vi "Dresden Edit Recipe(in).vi"() -> ()   [LabVIEW 2009] (continued)
            n1177 = local read "R Cmb Step3 Coating Power Active"() -> (w886:bool)
            n1178 = local read "R Cmb Step4 Coating Power Active"() -> (w885:bool)
            n1179 = local read "R Cmb Step5 Coating Power Active"() -> (w884:bool)
            n1180 = local read "R Cmb Step6 Coating Power Active"() -> (w883:bool)
            n1181 = local read "R Cmb Step7 Coating Power Active"() -> (w882:bool)
            n1182 = local read "R Cmb Step8 Coating Power Active"() -> (w881:bool)
            n1183 = local read "R Cmb Step9 Coating Power Active"() -> (w880:bool)
            n1184 = local read "R Cmb Step10 Coating Power Active"() -> (w879:bool)
            n1185 = local read "R Single RF Step6 Coating Power Active"() -> (w835:bool)
            n1186 = local read "R Cmb Interval length 1"() -> (w889:dbl)
            n1187 = Equal?(x=w1001, y=1) -> (x = y?=w999:bool)
            n1188 = case shown="False" w999 {
              frame #0 {
                w2466 = T5."Disabled and Grayed Out" ("Disabled")
                w2467 = 0.0 ("R Cmb Ch2 DC Ignition Power")
                w2468 = FALSE ("R Cmb Ch2 DC Target Clean Power Active")
                w2469 = ""
                n1189 = local write "R Cmb Number of cycle"(w2467) -> ()
                n1190 = local write "R Cmb Interval length 6"(w2467) -> ()
                n1191 = local write "R Cmb Interval length 7"(w2467) -> ()
                n1192 = local write "R Cmb Interval length 8"(w2467) -> ()
                n1193 = local write "R Cmb Interval length 9"(w2467) -> ()
                n1194 = local write "R Cmb Interval length 10"(w2467) -> ()
                n1195 = local write "R Cmb Ch2 Step6 Coating Power"(w2467) -> ()
                n1196 = local write "R Cmb Ch2 Step7 Coating Power"(w2467) -> ()
                n1197 = local write "R Cmb Ch2 Step8 Coating Power"(w2467) -> ()
                n1198 = local write "R Cmb Ch2 Step9 Coating Power"(w2467) -> ()
                n1199 = local write "R Cmb Ch2 Step10 Coating Power"(w2467) -> ()
                n1200 = local write "R Cmb Interval length 6"(w2467) -> ()
                n1201 = local write "R Cmb Interval length 7"(w2467) -> ()
                n1202 = local write "R Cmb Interval length 8"(w2467) -> ()
                n1203 = local write "R Cmb Interval length 9"(w2467) -> ()
                n1204 = local write "R Cmb Interval length 10"(w2467) -> ()
                n1205 = local write "R Cmb Interval length 1"(w2467) -> ()
                n1206 = local write "R Cmb Interval length 2"(w2467) -> ()
                n1207 = local write "R Cmb Interval length 3"(w2467) -> ()
                n1208 = local write "R Cmb Interval length 4"(w2467) -> ()
                n1209 = local write "R Cmb Interval length 5"(w2467) -> ()
                n1210 = local write "R Cmb Interval length 2"(w2467) -> ()
                n1211 = local write "R Cmb Interval length 3"(w2467) -> ()
                n1212 = local write "R Cmb Interval length 4"(w2467) -> ()
                n1213 = local write "R Cmb Interval length 5"(w2467) -> ()
                n1214 = local write "R Cmb Ch2 Step1 Coating Power"(w2467) -> ()
                n1215 = local write "R Cmb Ch2 Step2 Coating Power"(w2467) -> ()
                n1216 = local write "R Cmb Ch2 Step3 Coating Power"(w2467) -> ()
                n1217 = local write "R Cmb Ch2 Step4 Coating Power"(w2467) -> ()
                n1218 = local write "R Cmb Ch2 Step5 Coating Power"(w2467) -> ()
                n1219 = local write "R Cmb Ch3 Step1 Coating Power"(w2467) -> ()
                n1220 = local write "R Cmb Step6 Coating Power Active"(w2468) -> ()
                n1221 = local write "R Cmb Step7 Coating Power Active"(w2468) -> ()
                n1222 = local write "R Cmb Step8 Coating Power Active"(w2468) -> ()
                n1223 = local write "R Cmb Step9 Coating Power Active"(w2468) -> ()
                n1224 = local write "R Cmb Step10 Coating Power Active"(w2468) -> ()
                n1225 = local write "R Cmb Step1 Coating Power Active"(w2468) -> ()
                n1226 = local write "R Cmb Step2 Coating Power Active"(w2468) -> ()
                n1227 = local write "R Cmb Step3 Coating Power Active"(w2468) -> ()
                n1228 = local write "R Cmb Step4 Coating Power Active"(w2468) -> ()
                n1229 = local write "R Cmb Step5 Coating Power Active"(w2468) -> ()
                n1230 = local write "R Cmb Ch2 Target material"(w2469) -> ()
                n1231 = local write "R Cmb Ch3 Target material"(w2469) -> ()
                n1232 = property on="R Cmb Number of cycle" class="DigNum (strict)"("DisabledEnum"=w2466) -> ()  [unwired: 2 in, 2 out]
                n1233 = property on="R Cmb Ch2 Step1 Coating Power" class="DigNum (strict)"("DisabledEnum"=w2466) -> ()  [unwired: 2 in, 2 out]
                n1234 = property on="R Cmb Ch2 Step2 Coating Power" class="DigNum (strict)"("DisabledEnum"=w2466) -> ()  [unwired: 2 in, 2 out]
                n1235 = property on="R Cmb Ch2 Step3 Coating Power" class="DigNum (strict)"("DisabledEnum"=w2466) -> ()  [unwired: 2 in, 2 out]
                n1236 = property on="R Cmb Ch2 Step4 Coating Power" class="DigNum (strict)"("DisabledEnum"=w2466) -> ()  [unwired: 2 in, 2 out]
                n1237 = property on="R Cmb Ch2 Step5 Coating Power" class="DigNum (strict)"("DisabledEnum"=w2466) -> ()  [unwired: 2 in, 2 out]
                n1238 = property on="R Cmb Ch2 Step6 Coating Power" class="DigNum (strict)"("DisabledEnum"=w2466) -> ()  [unwired: 2 in, 2 out]
                n1239 = property on="R Cmb Ch2 Step7 Coating Power" class="DigNum (strict)"("DisabledEnum"=w2466) -> ()  [unwired: 2 in, 2 out]
                n1240 = property on="R Cmb Ch2 Step8 Coating Power" class="DigNum (strict)"("DisabledEnum"=w2466) -> ()  [unwired: 2 in, 2 out]
                n1241 = property on="R Cmb Ch2 Step9 Coating Power" class="DigNum (strict)"("DisabledEnum"=w2466) -> ()  [unwired: 2 in, 2 out]
                n1242 = property on="R Cmb Ch2 Step10 Coating Power" class="DigNum (strict)"("DisabledEnum"=w2466) -> ()  [unwired: 2 in, 2 out]
                n1243 = property on="R Cmb Ch3 Step1 Coating Power" class="DigNum (strict)"("DisabledEnum"=w2466) -> ()  [unwired: 2 in, 2 out]
                n1244 = property on="R Cmb Ch3 Step2 Coating Power" class="DigNum (strict)"("DisabledEnum"=w2466) -> ()  [unwired: 2 in, 2 out]
                n1245 = property on="R Cmb Ch3 Step3 Coating Power" class="DigNum (strict)"("DisabledEnum"=w2466) -> ()  [unwired: 2 in, 2 out]
                n1246 = property on="R Cmb Ch3 Step4 Coating Power" class="DigNum (strict)"("DisabledEnum"=w2466) -> ()  [unwired: 2 in, 2 out]
                n1247 = property on="R Cmb Ch3 Step5 Coating Power" class="DigNum (strict)"("DisabledEnum"=w2466) -> ()  [unwired: 2 in, 2 out]
                n1248 = property on="R Cmb Ch3 Step6 Coating Power" class="DigNum (strict)"("DisabledEnum"=w2466) -> ()  [unwired: 2 in, 2 out]
                n1249 = property on="R Cmb Ch3 Step7 Coating Power" class="DigNum (strict)"("DisabledEnum"=w2466) -> ()  [unwired: 2 in, 2 out]
                n1250 = property on="R Cmb Ch3 Step8 Coating Power" class="DigNum (strict)"("DisabledEnum"=w2466) -> ()  [unwired: 2 in, 2 out]
                n1251 = property on="R Cmb Ch3 Step9 Coating Power" class="DigNum (strict)"("DisabledEnum"=w2466) -> ()  [unwired: 2 in, 2 out]
                n1252 = property on="R Cmb Ch3 Step10 Coating Power" class="DigNum (strict)"("DisabledEnum"=w2466) -> ()  [unwired: 2 in, 2 out]
                n1253 = property on="R Cmb Interval length 10" class="DigNum (strict)"("DisabledEnum"=w2466) -> ()  [unwired: 2 in, 2 out]
                n1254 = property on="R Cmb Interval length 6" class="DigNum (strict)"("DisabledEnum"=w2466) -> ()  [unwired: 2 in, 2 out]
                n1255 = property on="R Cmb Interval length 7" class="DigNum (strict)"("DisabledEnum"=w2466) -> ()  [unwired: 2 in, 2 out]
                n1256 = property on="R Cmb Interval length 8" class="DigNum (strict)"("DisabledEnum"=w2466) -> ()  [unwired: 2 in, 2 out]
                n1257 = property on="R Cmb Interval length 9" class="DigNum (strict)"("DisabledEnum"=w2466) -> ()  [unwired: 2 in, 2 out]
                n1258 = property on="R Cmb Interval length 1" class="DigNum (strict)"("DisabledEnum"=w2466) -> ()  [unwired: 2 in, 2 out]
                n1259 = property on="R Cmb Interval length 2" class="DigNum (strict)"("DisabledEnum"=w2466) -> ()  [unwired: 2 in, 2 out]
                n1260 = property on="R Cmb Interval length 3" class="DigNum (strict)"("DisabledEnum"=w2466) -> ()  [unwired: 2 in, 2 out]
                n1261 = property on="R Cmb Interval length 4" class="DigNum (strict)"("DisabledEnum"=w2466) -> ()  [unwired: 2 in, 2 out]
                n1262 = property on="R Cmb Interval length 5" class="DigNum (strict)"("DisabledEnum"=w2466) -> ()  [unwired: 2 in, 2 out]
              }
              frame #1 {
                w2471 = T5."Disabled and Grayed Out" ("Disabled")
                n1263 = property on="R Single DC Interval length1" class="DigNum (strict)"("DisabledEnum"=w2471) -> ()  [unwired: 2 in, 2 out]
                n1264 = property on="R Single DC Step1 Coating Power" class="DigNum (strict)"("DisabledEnum"=w2471) -> ()  [unwired: 2 in, 2 out]
                n1265 = property on="R Cmb Number of cycle" class="DigNum (strict)"("DisabledEnum"=T5."Enabled" ("Disabled")) -> ()  [unwired: 2 in, 2 out]
                n1266 = local write "R Single DC Step1 Coating Power Active"(FALSE ("R Single DC Step1 Coating Power Active")) -> ()
                n1267 = local write "R Cmb Step1 Coating Power Active"(TRUE ("R Cmb Ch2 Step1 Coating Power Active")) -> ()
                n1268 = property on="R Single DC Target material" class="Str"("DisabledEnum"=T5."Disabled and Grayed Out" ("Disabled")) -> ()  [unwired: 2 in, 2 out]
              }
            }
            n1269 = case shown="True" w1011 {
              frame #0 {
                w2495 = T5."Disabled and Grayed Out" ("Disabled")
                w2494 = 0.0 ("R DC Ignition Power")
                w2493 = FALSE ("R DC Target Clean")
                n1270 = local write "R Single RF Interval length10"(w2494) -> ()
                n1271 = local write "R Single RF Interval length"(w2494) -> ()
                n1272 = local write "R Single RF Ramp up Time"(w2494) -> ()
                n1273 = local write "R Single RF  Step1 Coating Power"(w2494) -> ()
                n1274 = local write "R Single RF Step2 Coating Power"(w2494) -> ()
                n1275 = local write "R Single RF Step3 Coating Power"(w2494) -> ()
                n1276 = local write "R Single RF Step4 Coating Power"(w2494) -> ()
                n1277 = local write "R Single RF Step5 Coating Power"(w2494) -> ()
                n1278 = local write "R Single RF Ramp down Time"(w2494) -> ()
                n1279 = local write "R Single RF Interval length9"(w2494) -> ()
                n1280 = local write "R Single RF Interval length6"(w2494) -> ()
                n1281 = local write "R Single RF Target material"("") -> ()
                n1282 = local write "R Single RF Ramp up"(w2493) -> ()
                n1283 = local write "R Single RF Ramp down"(w2493) -> ()
                n1284 = local write "R Single RF Step1 Coating Power Active"(w2493) -> ()
                n1285 = local write "R Single RF Step2 Coating Power Active"(w2493) -> ()
                n1286 = local write "R Single RF Step3 Coating Power Active"(w2493) -> ()
                n1287 = local write "R Single RF Step4 Coating Power Active"(w2493) -> ()
                n1288 = local write "R Single RF Step5 Coating Power Active"(w2493) -> ()
                n1289 = local write "R Single RF Interval length8"(w2494) -> ()
                n1290 = local write "R Single RF Interval length7"(w2494) -> ()
                n1291 = local write "R Single RF Step6 Coating Power"(w2494) -> ()
                n1292 = local write "R Single RF Step7 Coating Power"(w2494) -> ()
                n1293 = local write "R Single RF Step8 Coating Power"(w2494) -> ()
                n1294 = local write "R Single RF Step9 Coating Power"(w2494) -> ()
                n1295 = local write "R Single RF Step10 Coating Power"(w2494) -> ()
                n1296 = local write "R Single RF Interval length2"(w2494) -> ()
                n1297 = local write "R Single RF Interval length3"(w2494) -> ()
                n1298 = local write "R Single RF Interval length4"(w2494) -> ()
                n1299 = local write "R Single RF Interval length5"(w2494) -> ()
                n1300 = local write "R Single RF Step6 Coating Power Active"(w2493) -> ()
                n1301 = local write "R Single RF Step7 Coating Power Active"(w2493) -> ()
                n1302 = local write "R Single RF Step8 Coating Power Active"(w2493) -> ()
                n1303 = local write "R Single RF Step9 Coating Power Active"(w2493) -> ()
                n1304 = local write "R Single RF Step10 Coating Power Active"(w2493) -> ()
                n1305 = property on="R Single RF Interval length" class="DigNum (strict)"("DisabledEnum"=w2495) -> ()  [unwired: 2 in, 2 out]
                n1306 = property on="R Single RF Step6 Coating Power" class="DigNum (strict)"("DisabledEnum"=w2495) -> ()  [unwired: 2 in, 2 out]
                n1307 = property on="R Single RF Step7 Coating Power" class="DigNum (strict)"("DisabledEnum"=w2495) -> ()  [unwired: 2 in, 2 out]
                n1308 = property on="R Single RF Step8 Coating Power" class="DigNum (strict)"("DisabledEnum"=w2495) -> ()  [unwired: 2 in, 2 out]
                n1309 = property on="R Single RF Step9 Coating Power" class="DigNum (strict)"("DisabledEnum"=w2495) -> ()  [unwired: 2 in, 2 out]
                n1310 = property on="R Single RF Step10 Coating Power" class="DigNum (strict)"("DisabledEnum"=w2495) -> ()  [unwired: 2 in, 2 out]
                n1311 = property on="R Single RF Interval length2" class="DigNum (strict)"("DisabledEnum"=w2495) -> ()  [unwired: 2 in, 2 out]
                n1312 = property on="R Single RF Interval length3" class="DigNum (strict)"("DisabledEnum"=w2495) -> ()  [unwired: 2 in, 2 out]
                n1313 = property on="R Single RF Interval length4" class="DigNum (strict)"("DisabledEnum"=w2495) -> ()  [unwired: 2 in, 2 out]
                n1314 = property on="R Single RF Interval length5" class="DigNum (strict)"("DisabledEnum"=w2495) -> ()  [unwired: 2 in, 2 out]
                n1315 = property on="R Single RF Interval length6" class="DigNum (strict)"("DisabledEnum"=w2495) -> ()  [unwired: 2 in, 2 out]
                n1316 = property on="R Single RF Ramp up Time" class="DigNum (strict)"("DisabledEnum"=w2495) -> ()  [unwired: 2 in, 2 out]
                n1317 = property on="R Single RF  Step1 Coating Power" class="DigNum (strict)"("DisabledEnum"=w2495) -> ()  [unwired: 2 in, 2 out]
                n1318 = property on="R Single RF Step2 Coating Power" class="DigNum (strict)"("DisabledEnum"=w2495) -> ()  [unwired: 2 in, 2 out]
                n1319 = property on="R Single RF Step3 Coating Power" class="DigNum (strict)"("DisabledEnum"=w2495) -> ()  [unwired: 2 in, 2 out]
                n1320 = property on="R Single RF Step4 Coating Power" class="DigNum (strict)"("DisabledEnum"=w2495) -> ()  [unwired: 2 in, 2 out]
                n1321 = property on="R Single RF Step5 Coating Power" class="DigNum (strict)"("DisabledEnum"=w2495) -> ()  [unwired: 2 in, 2 out]
                n1322 = property on="R Single RF Ramp down Time" class="DigNum (strict)"("DisabledEnum"=w2495) -> ()  [unwired: 2 in, 2 out]
                n1323 = property on="R Single RF Interval length10" class="DigNum (strict)"("DisabledEnum"=w2495) -> ()  [unwired: 2 in, 2 out]
                n1324 = property on="R Single RF Interval length9" class="DigNum (strict)"("DisabledEnum"=w2495) -> ()  [unwired: 2 in, 2 out]
                n1325 = property on="R Single RF Interval length7" class="DigNum (strict)"("DisabledEnum"=w2495) -> ()  [unwired: 2 in, 2 out]
                n1326 = property on="R Single RF Interval length8" class="DigNum (strict)"("DisabledEnum"=w2495) -> ()  [unwired: 2 in, 2 out]
              }
              frame #1 {
                n1327 = local write "R Single RF Step1 Coating Power Active"(TRUE ("R Single RF Step1 Coating Power Active")) -> ()
                n1328 = local write "R Set Pressure mtorr"(0.001 ("R Set Pressure mtorr")) -> ()
              }
            }
            n1329 = local read "R Single DC Step5 Coating Power Active"() -> (w846:bool)
            n1330 = case shown="True" w1016 {
              frame #0 {
                w2499 = 0.0 ("R_Microwave Power")
                w2500 = T5."Enabled" ("Disabled")
                n1331 = property on="R Argon Flow sccm" class="DigNum (strict)"("DisabledEnum"=w2500) -> ()  [unwired: 2 in, 2 out]
                n1332 = property on="R Set Pressure mtorr" class="DigNum (strict)"("DisabledEnum"=w2500) -> ()  [unwired: 2 in, 2 out]
                n1333 = local write "R_Single Microwave Power"(w2499) -> ()
                n1334 = local write "R_Single Microwave Time"(w2499) -> ()
                n1335 = property on="R_Single Microwave Power" class="DigNum (strict)"("DisabledEnum"=T5."Disabled and Grayed Out" ("Disabled")) -> ()  [unwired: 2 in, 2 out]
                n1336 = local write "R Single Pass Number"(w2499) -> ()
              }
              frame #1 {
                w2509 = T5."Disabled and Grayed Out" ("Disabled")
                n1337 = property on="R Set Pressure mtorr" class="DigNum (strict)"("DisabledEnum"=w2509) -> ()  [unwired: 2 in, 2 out]
                n1338 = property on="R Argon Flow sccm" class="DigNum (strict)"("DisabledEnum"=w2509) -> ()  [unwired: 2 in, 2 out]
                n1339 = local read "R Single Pass Number"() -> (w2507:dbl)
                n1340 = property on="R_Single Microwave Power" class="DigNum (strict)"("DisabledEnum"=T5."Enabled" ("Disabled")) -> ()  [unwired: 2 in, 2 out]
                n1341 = local write "R Argon Flow sccm"(200.0 ("R Argon Flow sccm")) -> ()
                n1342 = local write "R Set Pressure mtorr"(0.011 ("R Set Pressure mtorr")) -> ()
                n1343 = Less Or Equal?(x=w2507, y=1.5) -> (x <= y?=w2505:bool)
                n1344 = Select(t=1, s=w2505, f=2) -> (s? t:f=w2502:i32)
                n1345 = local write "R Single Pass Number"(w2502) -> ()
              }
            }
            n1346 = case shown="True" w1013 {
              frame #0 {
                w2487 = T5."Disabled and Grayed Out" ("Disabled")
                w2488 = 0.0 ("R DC Ignition Power")
                w2489 = FALSE ("R DC Target Clean")
                n1347 = local write "R Single DC Step1 Coating Power Active"(w2489) -> ()
                n1348 = local write "R Single DC Step2 Coating Power Active"(w2489) -> ()
                n1349 = local write "R Single DC Step3 Coating Power Active"(w2489) -> ()
                n1350 = local write "R Single DC Step4 Coating Power Active"(w2489) -> ()
                n1351 = local write "R Single DC Step5 Coating Power Active"(w2489) -> ()
                n1352 = local write "R Single DC Step6 Coating Power Active"(w2489) -> ()
                n1353 = local write "R Single DC Step7 Coating Power Active"(w2489) -> ()
                n1354 = local write "R Single DC Step8 Coating Power Active"(w2489) -> ()
                n1355 = local write "R Single DC Step9 Coating Power Active"(w2489) -> ()
                n1356 = local write "R Single DC Step10 Coating Power Active"(w2489) -> ()
                n1357 = local write "R_Single DC_Material ok"(w2489) -> ()
                n1358 = local write "R Single DC Target material"("") -> ()
                n1359 = local write "R Single DC Interval length1"(w2488) -> ()
                n1360 = local write "R Single DC Step1 Coating Power"(w2488) -> ()
                n1361 = local write "R Single DC Step2 Coating Power"(w2488) -> ()
                n1362 = local write "R Single DC Step3 Coating Power"(w2488) -> ()
                n1363 = local write "R Single DC Step4 Coating Power"(w2488) -> ()
                n1364 = local write "R Single DC Step5 Coating Power"(w2488) -> ()
                n1365 = local write "R Single DC Interval length2"(w2488) -> ()
                n1366 = local write "R Single DC Interval length3"(w2488) -> ()
                n1367 = local write "R Single DC Interval length4"(w2488) -> ()
                n1368 = local write "R Single DC Interval length5"(w2488) -> ()
                n1369 = local write "R Single DC Interval length6"(w2488) -> ()
                n1370 = local write "R Single DC Interval length7"(w2488) -> ()
                n1371 = local write "R Single DC Interval length8"(w2488) -> ()
                n1372 = local write "R Single DC Interval length9"(w2488) -> ()
                n1373 = local write "R Single DC Interval length10"(w2488) -> ()
                n1374 = property on="R Single DC Step6 Coating Power" class="DigNum (strict)"("DisabledEnum"=w2487) -> ()  [unwired: 2 in, 2 out]
                n1375 = property on="R Single DC Step7 Coating Power" class="DigNum (strict)"("DisabledEnum"=w2487) -> ()  [unwired: 2 in, 2 out]
                n1376 = property on="R Single DC Interval length6" class="DigNum (strict)"("DisabledEnum"=w2487) -> ()  [unwired: 2 in, 2 out]
                n1377 = property on="R Single DC Step1 Coating Power" class="DigNum (strict)"("DisabledEnum"=w2487) -> ()  [unwired: 2 in, 2 out]
                n1378 = property on="R Single DC Step2 Coating Power" class="DigNum (strict)"("DisabledEnum"=w2487) -> ()  [unwired: 2 in, 2 out]
                n1379 = property on="R Single DC Step3 Coating Power" class="DigNum (strict)"("DisabledEnum"=w2487) -> ()  [unwired: 2 in, 2 out]
                n1380 = property on="R Single DC Step4 Coating Power" class="DigNum (strict)"("DisabledEnum"=w2487) -> ()  [unwired: 2 in, 2 out]
                n1381 = property on="R Single DC Step5 Coating Power" class="DigNum (strict)"("DisabledEnum"=w2487) -> ()  [unwired: 2 in, 2 out]
                n1382 = property on="R Single DC Interval length1" class="DigNum (strict)"("DisabledEnum"=w2487) -> ()  [unwired: 2 in, 2 out]
                n1383 = property on="R Single DC Step8 Coating Power" class="DigNum (strict)"("DisabledEnum"=w2487) -> ()  [unwired: 2 in, 2 out]
                n1384 = property on="R Single DC Step9 Coating Power" class="DigNum (strict)"("DisabledEnum"=w2487) -> ()  [unwired: 2 in, 2 out]
                n1385 = property on="R Single DC Step10 Coating Power" class="DigNum (strict)"("DisabledEnum"=w2487) -> ()  [unwired: 2 in, 2 out]
                n1386 = property on="R Single DC Interval length2" class="DigNum (strict)"("DisabledEnum"=w2487) -> ()  [unwired: 2 in, 2 out]
                n1387 = property on="R Single DC Interval length3" class="DigNum (strict)"("DisabledEnum"=w2487) -> ()  [unwired: 2 in, 2 out]
                n1388 = property on="R Single DC Interval length4" class="DigNum (strict)"("DisabledEnum"=w2487) -> ()  [unwired: 2 in, 2 out]
                n1389 = property on="R Single DC Interval length5" class="DigNum (strict)"("DisabledEnum"=w2487) -> ()  [unwired: 2 in, 2 out]
                n1390 = property on="R Single DC Interval length7" class="DigNum (strict)"("DisabledEnum"=w2487) -> ()  [unwired: 2 in, 2 out]
                n1391 = property on="R Single DC Interval length6" class="DigNum (strict)"("DisabledEnum"=w2487) -> ()  [unwired: 2 in, 2 out]
                n1392 = property on="R Single DC Interval length8" class="DigNum (strict)"("DisabledEnum"=w2487) -> ()  [unwired: 2 in, 2 out]
                n1393 = property on="R Single DC Interval length9" class="DigNum (strict)"("DisabledEnum"=w2487) -> ()  [unwired: 2 in, 2 out]
                n1394 = property on="R Single DC Interval length10" class="DigNum (strict)"("DisabledEnum"=w2487) -> ()  [unwired: 2 in, 2 out]
              }
              frame #1 {
                n1395 = local write "R Single DC Step1 Coating Power Active"(TRUE ("R Single DC Step1 Coating Power Active")) -> ()
                n1396 = local write "R Set Pressure mtorr"(0.004 ("R Set Pressure mtorr")) -> ()
              }
            }
            n1397 = local read "R Single RF Step7 Coating Power Active"() -> (w834:bool)
            n1398 = local read "R Single DC Step6 Coating Power Active"() -> (w845:bool)
            n1399 = Boolean To (0,1)(Boolean=w890) -> (0, 1=w900:i16)
            n1400 = case shown="False" w842 {
              frame #0 {
                n1401 = local write "R Single DC Step10 Coating Power Active"(FALSE ("R Single DC Step8 Coating Power Active")) -> ()
              }
              frame #1 {
                n1402 = local read "R Single DC Step10 Coating Power Active"() -> (w1118:bool)
                n1403 = case shown="False" w1118 {
                  frame #0 {
                    w1119 = 0.0 ("R Single DC Step10 Coating Power")
                    w1120 = T5."Disabled and Grayed Out" ("Disabled")
                    n1404 = local write "R Single DC Step10 Coating Power"(w1119) -> ()
                    n1405 = local write "R Single DC Interval length10"(w1119) -> ()
                    n1406 = property on="R Single DC Step10 Coating Power" class="DigNum (strict)"("DisabledEnum"=w1120) -> ()  [unwired: 2 in, 2 out]
                    n1407 = property on="R Single DC Interval length10" class="DigNum (strict)"("DisabledEnum"=w1120) -> ()  [unwired: 2 in, 2 out]
                  }
                  frame #1 {
                    w1121 = T5."Enabled" ("Disabled")
                    n1408 = property on="R Single DC Step10 Coating Power" class="DigNum (strict)"("DisabledEnum"=w1121) -> ()  [unwired: 2 in, 2 out]
                    n1409 = property on="R Single DC Interval length10" class="DigNum (strict)"("DisabledEnum"=w1121) -> ()  [unwired: 2 in, 2 out]
                  }
                }
              }
            }
            n1410 = case shown="False" w843 {
              frame #0 {
                w1122 = FALSE ("R Single DC Step8 Coating Power Active")
                n1411 = local write "R Single DC Step10 Coating Power Active"(w1122) -> ()
                n1412 = local write "R Single DC Step9 Coating Power Active"(w1122) -> ()
              }
              frame #1 {
                n1413 = local read "R Single DC Step9 Coating Power Active"() -> (w1123:bool)
                n1414 = case shown="False" w1123 {
                  frame #0 {
                    w1124 = 0.0 ("R Single DC Step9 Coating Power")
                    w1125 = T5."Disabled and Grayed Out" ("Disabled")
                    n1415 = property on="R Single DC Step9 Coating Power" class="DigNum (strict)"("DisabledEnum"=w1125) -> ()  [unwired: 2 in, 2 out]
                    n1416 = property on="R Single DC Interval length9" class="DigNum (strict)"("DisabledEnum"=w1125) -> ()  [unwired: 2 in, 2 out]
                    n1417 = local write "R Single DC Step9 Coating Power"(w1124) -> ()
                    n1418 = local write "R Single DC Interval length9"(w1124) -> ()
                  }
                  frame #1 {
                    w1126 = T5."Enabled" ("Disabled")
                    n1419 = property on="R Single DC Interval length9" class="DigNum (strict)"("DisabledEnum"=w1126) -> ()  [unwired: 2 in, 2 out]
                    n1420 = property on="R Single DC Step9 Coating Power" class="DigNum (strict)"("DisabledEnum"=w1126) -> ()  [unwired: 2 in, 2 out]
                  }
                }
              }
            }
            n1421 = local read "R Cmb Interval length 9"() -> (w872:dbl)
            n1422 = local read "R Cmb Interval length 3"() -> (w878:dbl)
            n1423 = local read "R Cmb Interval length 4"() -> (w877:dbl)
            n1424 = local read "R Cmb Interval length 10"() -> (w871:dbl)
            n1425 = local read "R Cmb Interval length 2"() -> (w887:dbl)
            n1426 = local read "R Cmb Interval length 5"() -> (w876:dbl)
            n1427 = case shown="True" w988 {
              frame #0 {
                w1951 = T5."Disabled and Grayed Out" ("Disabled")
                n1428 = property on="R Material_density" class="DigNum (strict)"("DisabledEnum"=w1951) -> ()  [unwired: 2 in, 2 out]
                n1429 = property on="R Z_factor" class="DigNum (strict)"("DisabledEnum"=w1951) -> ()  [unwired: 2 in, 2 out]
                n1430 = property on="R Toooling_factor" class="DigNum (strict)"("DisabledEnum"=w1951) -> ()  [unwired: 2 in, 2 out]
              }
              frame #1 {
                w1952 = T5."Enabled" ("Disabled")
                n1431 = property on="R Material_density" class="DigNum (strict)"("DisabledEnum"=w1952) -> ()  [unwired: 2 in, 2 out]
                n1432 = property on="R Z_factor" class="DigNum (strict)"("DisabledEnum"=w1952) -> ()  [unwired: 2 in, 2 out]
                n1433 = property on="R Toooling_factor" class="DigNum (strict)"("DisabledEnum"=w1952) -> ()  [unwired: 2 in, 2 out]
              }
            }
            n1434 = local read "R Cmb Interval length 6"() -> (w874:dbl)
            n1435 = local read "R Cmb Interval length 8"() -> (w873:dbl)
            n1436 = local read "R Cmb Interval length 7"() -> (w875:dbl)
            n1437 = Multiply(x=w900, y=w889) -> (x*y=w869:dbl)
            n1438 = local read "R Single DC Step7 Coating Power Active"() -> (w844:bool)
            n1439 = Boolean To (0,1)(Boolean=w888) -> (0, 1=w899:i16)
            n1440 = Boolean To (0,1)(Boolean=w886) -> (0, 1=w898:i16)
            n1441 = Boolean To (0,1)(Boolean=w885) -> (0, 1=w897:i16)
            n1442 = Boolean To (0,1)(Boolean=w883) -> (0, 1=w895:i16)
            n1443 = Boolean To (0,1)(Boolean=w881) -> (0, 1=w893:i16)
            n1444 = Boolean To (0,1)(Boolean=w884) -> (0, 1=w896:i16)
            n1445 = Boolean To (0,1)(Boolean=w880) -> (0, 1=w892:i16)
            n1446 = Boolean To (0,1)(Boolean=w879) -> (0, 1=w891:i16)
            n1447 = Boolean To (0,1)(Boolean=w882) -> (0, 1=w894:i16)
            n1448 = case shown="False" w835 {
              frame #0 {
                w1083 = FALSE ("R Single RF Step3 Coating Power Active")
                n1449 = local write "R Single RF Step7 Coating Power Active"(w1083) -> ()
                n1450 = local write "R Single RF Step8 Coating Power Active"(w1083) -> ()
                n1451 = local write "R Single RF Step9 Coating Power Active"(w1083) -> ()
                n1452 = local write "R Single RF Step10 Coating Power Active"(w1083) -> ()
              }
              frame #1 {
                n1453 = local read "R Single RF Step7 Coating Power Active"() -> (w1084:bool)
                n1454 = case shown="False" w1084 {
                  frame #0 {
                    w1085 = 0.0 ("Target Clean Power")
                    w1086 = T5."Disabled and Grayed Out" ("Disabled")
                    n1455 = local write "R Single RF Step7 Coating Power"(w1085) -> ()
                    n1456 = local write "R Single RF Interval length7"(w1085) -> ()
                    n1457 = property on="R Single RF Step7 Coating Power" class="DigNum (strict)"("DisabledEnum"=w1086) -> ()  [unwired: 2 in, 2 out]
                    n1458 = property on="R Single RF Interval length7" class="DigNum (strict)"("DisabledEnum"=w1086) -> ()  [unwired: 2 in, 2 out]
                  }
                  frame #1 {
                    w1087 = T5."Enabled" ("Disabled")
                    n1459 = property on="R Single RF Step7 Coating Power" class="DigNum (strict)"("DisabledEnum"=w1087) -> ()  [unwired: 2 in, 2 out]
                    n1460 = property on="R Single RF Interval length7" class="DigNum (strict)"("DisabledEnum"=w1087) -> ()  [unwired: 2 in, 2 out]
                  }
                }
              }
            }
            n1461 = Multiply(x=w899, y=w887) -> (x*y=w868:dbl)
            n1462 = Multiply(x=w898, y=w878) -> (x*y=w867:dbl)
            n1463 = Multiply(x=w897, y=w877) -> (x*y=w866:dbl)
            n1464 = case shown="False" w834 {
              frame #0 {
                w1078 = FALSE ("R Single RF Step3 Coating Power Active")
                n1465 = local write "R Single RF Step8 Coating Power Active"(w1078) -> ()
                n1466 = local write "R Single RF Step9 Coating Power Active"(w1078) -> ()
                n1467 = local write "R Single RF Step10 Coating Power Active"(w1078) -> ()
              }
              frame #1 {
                n1468 = local read "R Single RF Step8 Coating Power Active"() -> (w1079:bool)
                n1469 = case shown="False" w1079 {
                  frame #0 {
                    w1080 = 0.0 ("Target Clean Power")
                    w1081 = T5."Disabled and Grayed Out" ("Disabled")
                    n1470 = local write "R Single RF Step8 Coating Power"(w1080) -> ()
                    n1471 = local write "R Single RF Interval length8"(w1080) -> ()
